vi "kinectRead [BodyFrame].vi"(8 "error in (no error)":errorcluster, 10 "Wrapper Reference":refnum<k24>, 11 "KinectSensor References in":T2) -> (0 "error out":errorcluster, 2 "Body Data":T1[](array[typedef]) {"LeanTrackingState" items=["NotTracked", "Inferred", "Tracked"]; "HandRightState" items=["Unknown", "NotTracked", "Open", "Closed", "Lasso"]; "HandRightConfidence" items=["Low", "High"]; "HandLeftState" items=["Unknown", "NotTracked", "Open", "Closed", "Lasso"]; "HandLeftConfidence" items=["Low", "High"]; "ClippedEdges" items=["None"=0, "Right"=1, "Left"=2, "Top"=4, "Bottom"=8]}, 3 "KinectSensor References out":T2)   [LabVIEW 2014]
uses:
  controls/KinectSensor References.ctl
  Microsoft.Kinect
  C:/Users/iknox/Documents/Visual Studio 2013/Projects/ConvertListToArray/ConvertListToArray/ClassLibrary1/bin/Debug/ListToArrayWrapper.dll
  Users/iknox/Documents/Visual Studio 2013/Projects/ConvertListToArray/ConvertListToArray/ClassLibrary1/bin/Debug/ListToArrayWrapper.dll
  controls/BodyData.ctl
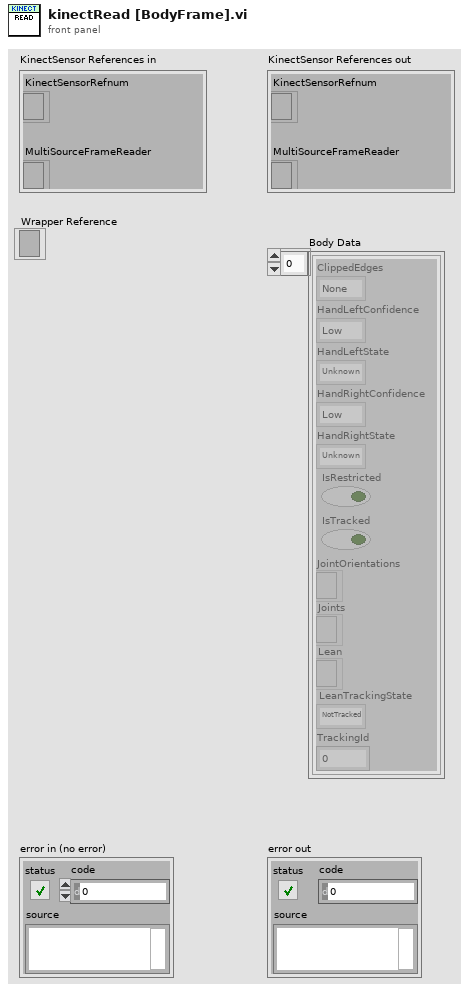
[diagram p1: front panel]
types:
  T1 = typedef "BodyData.ctl" = cluster{"ClippedEdges":i32, "HandLeftConfidence":i32, "HandLeftState":i32, "HandRightConfidence":i32, "HandRightState":i32, "IsRestricted":bool, "IsTracked":bool, "JointOrientations":refnum<k24>, "Joints":refnum<k24>, "Lean":refnum<k24>, "LeanTrackingState":i32, "TrackingId":u64}
  T2 = typedef "KinectSensor References.ctl" = cluster{"KinectSensorRefnum":refnum<k24>, "MultiSourceFrameReader":refnum<k24>}
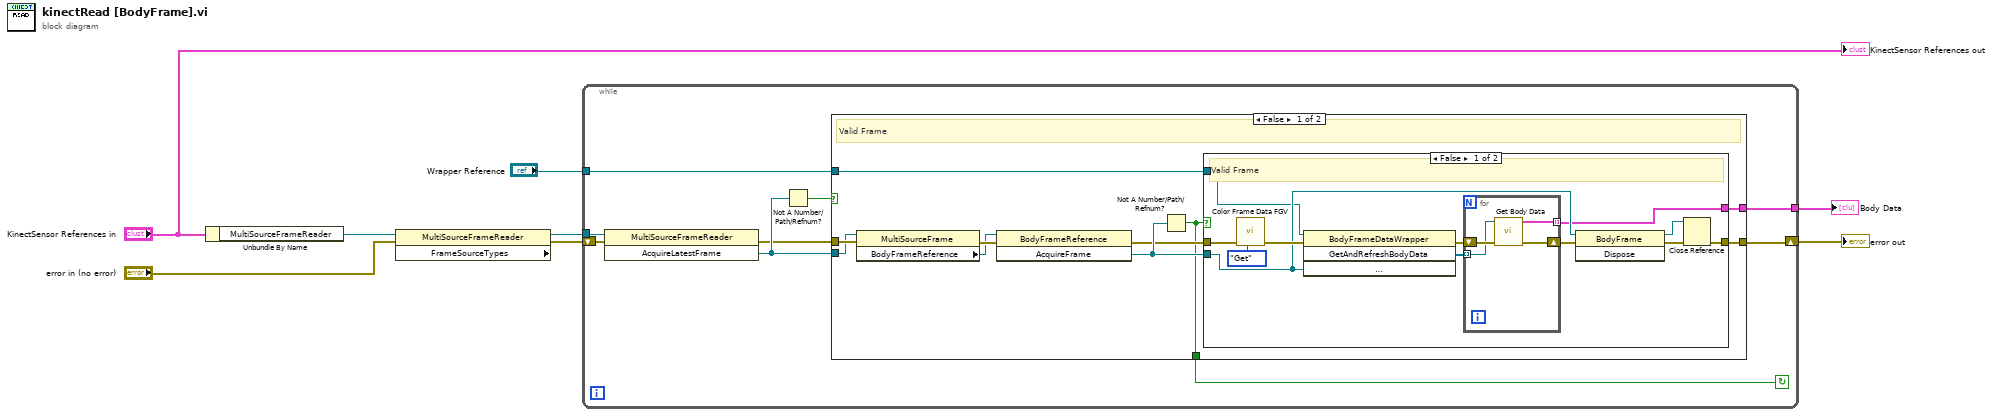
[diagram p0: block diagram]
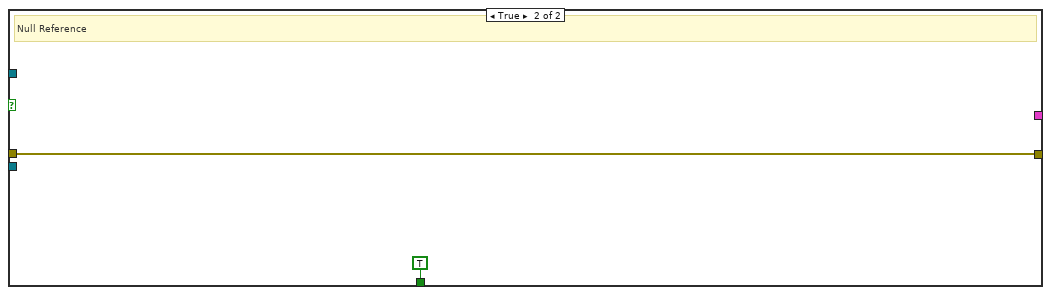
[diagram p3: hidden frame]
diagram:
  n1 = Unbundle By Name("KinectSensor References in") -> ("MultiSourceFrameReader"=w6:refnum<k24>)
  n2 = property class="MultiSourceFrameReader" props=["FrameSourceTypes"](reference=w6, error in="error in (no error)") -> (reference out=w8:refnum<k24>, error out=w7:errorcluster)  [unwired: 1 out]
  n3 = while {
    tunnel: w8 -> [w17]
    shift-right: [w12] -> w3
    shift-left: w7 -> [w16]
    tunnel: "Wrapper Reference" -> [w10]
    tunnel: [w9] -> w1
    stop <- w11 continue-if-true
    n4 = invoke class="MultiSourceFrameReader" method="AcquireLatestFrame"(reference=w17, error in=w16) -> (error out=w14:errorcluster, "AcquireLatestFrame"=w15:refnum<k24>)  [unwired: 1 in, 1 out]
    n5 = Not A Number/Path/Refnum?(number/path/refnum=w15) -> (NaN/Path/Refnum?=w13:bool)
    n6 = case shown="False" w13 {
      tunnel: w14 -> [w24 w45]
      tunnel: w15 -> [w21 _]
      tunnel: [w23 w45] -> w12
      tunnel: [w22 TRUE] -> w11
      tunnel: w10 -> [w19 _]
      tunnel: [w18 _] -> w9
      frame False {
        # "Valid Frame"
        n7 = property class="MultiSourceFrame"(reference=w21, error in=w24) -> (error out=w25:errorcluster, "BodyFrameReference"=w20:refnum<k24>)  [unwired: 1 out]
        n8 = invoke class="BodyFrameReference" method="AcquireFrame"(reference=w20, error in=w25) -> (error out=w26:errorcluster, "AcquireFrame"=w27:refnum<k24>)  [unwired: 1 in, 1 out]
        n9 = Not A Number/Path/Refnum?(number/path/refnum=w27) -> (NaN/Path/Refnum?=w22:bool)
        n10 = case shown="False" w22 {
          tunnel: w26 -> [w36 w44]
          tunnel: w27 -> [w31 _]
          tunnel: [w35 w44] -> w23
          tunnel: w19 -> [w29 _]
          tunnel: [w28 _] -> w18
          frame False {
            # "Valid Frame"
            n11 = call "Color Frame Data FGV.vi"("Command"=enum16{"Get", "Initialize"}."Get", "error in (no error)"=w36) -> ("error out"=w34:errorcluster)  [unwired: 8 in, 1 out]
            n12 = invoke class="BodyFrameDataWrapper" method="GetAndRefreshBodyData"(reference=w29, error in=w34, "bodyFrame"=w31) -> (error out=w32:errorcluster, "GetAndRefreshBodyData"=w33:refnum<k24>[])  [unwired: 1 in, 2 out]
            n13 = for {
              tunnel: w33 -> [w41] mode=indexing
              shift-right: [w42] -> w30
              shift-left: w32 -> [w43]
              tunnel: [w40] -> w28 mode=indexing
              n14 = call "Get Body Data.vi"("error in (no error)"=w43, "Body Reference"=w41) -> ("error out"=w42:errorcluster, "BodyData"=w40:T1)  [unwired: 8 in]
            }
            n15 = invoke class="BodyFrame" method="Dispose"(reference=w31, error in=w30) -> (reference out=w39:refnum<k24>, error out=w38:errorcluster)  [unwired: 1 in, 1 out]
            n16 = Close Reference(reference=w39, error in (no error)=w38) -> (error out=w35:errorcluster)
          }
          frame True {
            # "Null Reference"
          }
        }
      }
      frame True {
        # "Null Reference"
      }
    }
  }
  "error out" <- w3
  "Body Data" <- w1
  "KinectSensor References out" <- "KinectSensor References in"
